vi "Test Find Class located within Library.vi"(8 "error in (no error)":errorcluster, 11 "Test Finder Test in":refnum<class "Finder Test.lvclass">) -> (0 "error out":errorcluster, 3 "Test Finder Test out":refnum<class "Finder Test.lvclass">)   [LabVIEW 2020, in "LUnit Tests.lvlib" / "Finder Test.lvclass"]
uses:
  Finder Test.lvclass
  Finder Test.lvclass/Finder Test.ctl
  source/Framework/Helper Classes/Test Finder/Test Finder.lvclass
  <vilib>/Astemes/LUnit/Test Case.lvclass
  Test Dummys/Dummy Library/Test Test Case.lvclass
  C:/Program Files (x86)/National Instruments/LabVIEW 2020/vi.lib/Astemes/LUnit/Test Case.lvclass
  C:/Git/astemes-lunit/tests/Test Finder/Finder Test.lvclass
  C:/Git/astemes-lunit/source/Framework/Test Case/LUnit Test Case.lvclass
  C:/Git/astemes-lunit/tests/Test Dummys/Dummy Library/Test Test Case.lvclass
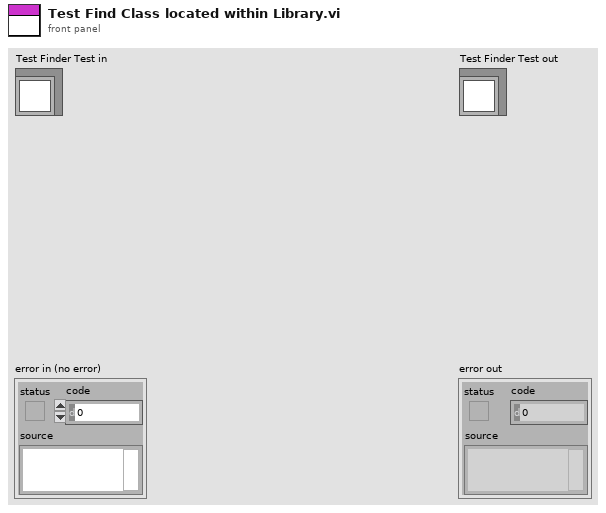
[diagram p1: front panel]
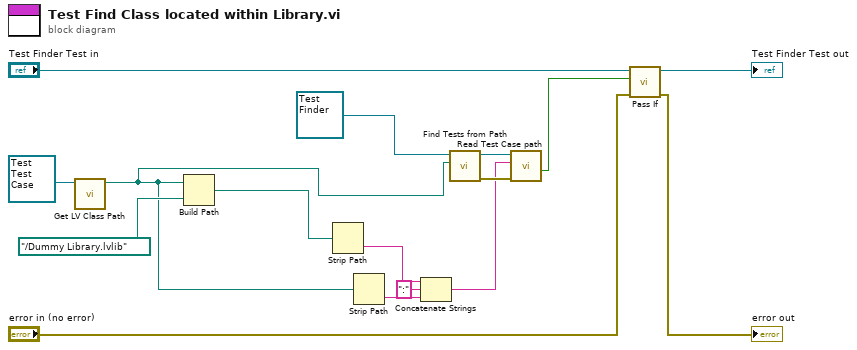
[diagram p0: block diagram]
diagram:
  n1 = call <vilib>:"Get LV Class Path.vi"("object"=refnum<class "Test Test Case.lvclass"> refnum ("Dummy Library.lvlib:Test Test Case.lvclass")) -> ("class path"=w2:path)  [unwired: 9 in, 1 out]
  n2 = Build Path(base path=w2, name or relative path=path "../Dummy Library.lvlib") -> (appended path=w1:path)
  n3 = Strip Path(path=w1) -> (name=w4:string)  [unwired: 1 out]
  n4 = Strip Path(path=w2) -> (name=w9:string)  [unwired: 1 out]
  n5 = Concatenate Strings(w4, ":" ("string"), w9) -> (w5:string)
  n6 = call-dynamic "Find Tests from Path.vi"("Project or Class Path"=w2, "Test Case Finder In"=refnum<class "Test Finder.lvclass"> refnum) -> ("error out"=w11:errorcluster, "Test Case Finder Out"=w12:refnum<class "Test Finder.lvclass">)  [unwired: 8 in]
  n7 = call "Read Test Case path.vi"("error in (no error)"=w11, "Test Case Name"=w5, "Test Case Finder In"=w12) -> ("found?"=w8:bool)  [unwired: 5 in, 3 out]
  n8 = call <vilib>:"Pass If.vi"("error in (no error)"="error in (no error)", "Pass?"=w8, "LUnit Test Case In"="Test Finder Test in") -> ("error out"=→"error out":errorcluster, "LUnit Test Case Out"=→"Test Finder Test out":refnum<class "Finder Test.lvclass">)  [unwired: 7 in]
